vi "AssertInvisible.vi"(0 "VI Reference In":refnum<vi>, 1 "Label":string, 2 "delimiter (>>)":string=">>", 3 "Assert Only? (F)":bool, 5 "Control Path":string, 11 "Error In":errorcluster, 12 "Assert Interval(10 ms)":u32=10, 13 "Timeout(5 sec)":dbl=5.0) -> (4 "VI Reference Out":refnum<vi>, 6 "Asserted Value":bool caption="Asserted Value (Visible ?)", 15 "Error Out":errorcluster)   [LabVIEW 2016, in "Drona.lvlib" / "AssertControlProperty.lvlib" / "AssertControlVisible.lvlib"]
doc: "Asserts if the control is invisible.\n\nThe input control name is given as a string , incase of path, use delimiters inbetween the path.\nThis VI checks until the control is insvisible."
uses:
  AssertControlVisible.lvlib
  Get/GetControlRef/GetControlRefByPath.vi
  <vilib>/addons/_JKI Toolkits/Caraya/classes/Assert/Assert False.vi
  <vilib>/addons/_JKI Toolkits/Caraya/classes/Assert/Assert.lvclass
  Get/GetControlRef/GetControlRef.lvlib
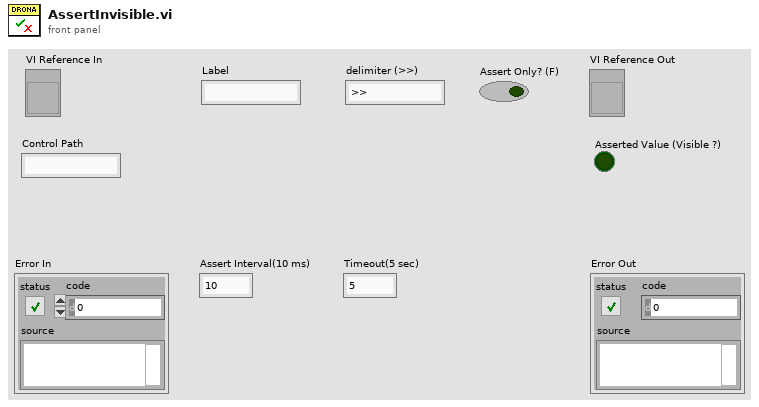
[diagram p1: front panel]
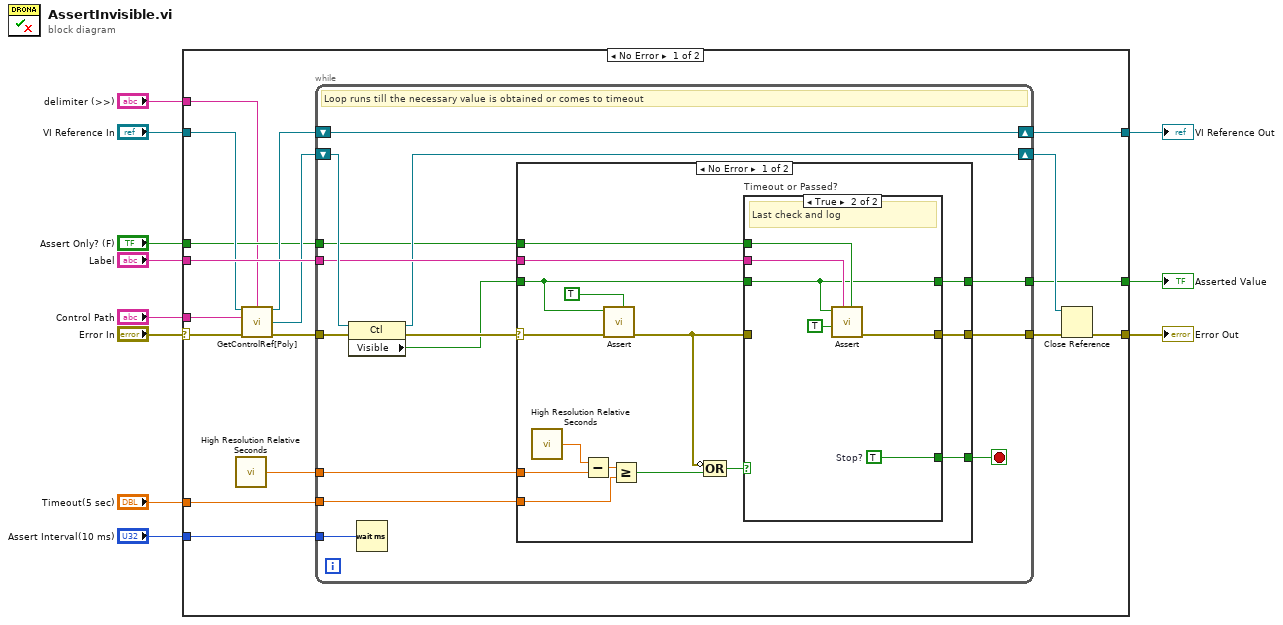
[diagram p0: block diagram]
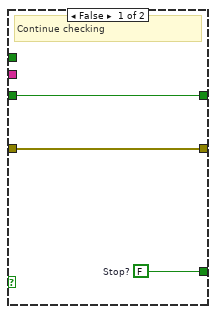
[diagram p2: hidden frame]
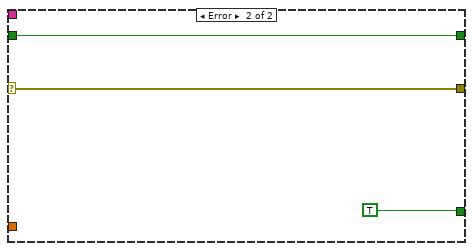
[diagram p3: hidden frame]
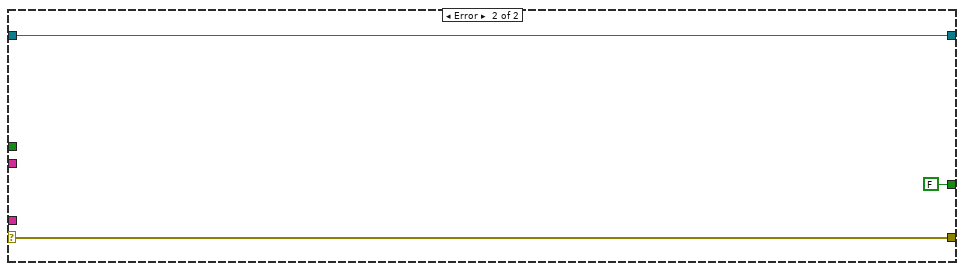
[diagram p4: hidden frame]
diagram:
  n1 = case shown="No Error" "Error In" {
    selector: "Error In" -> [w23 w72]
    tunnel: "Timeout(5 sec)" -> [w28 _]
    tunnel: [w27 w71] -> w10
    tunnel: [w17 w72] -> w9
    tunnel: "Assert Interval(10 ms)" -> [w25 _]
    tunnel: "Label" -> [w24 _]
    tunnel: "VI Reference In" -> [w22 w71]
    tunnel: "Control Path" -> [w12 _]
    tunnel: "delimiter (>>)" -> [w13 _]
    tunnel: "Assert Only? (F)" -> [w15 _]
    tunnel: [w14 FALSE ("Visible")] -> w1
    frame No Error {
      n2 = call <vilib>:"High Resolution Relative Seconds.vi"() -> ("relative seconds"=w21:dbl)
      n3 = call-poly "GetControlRef[Poly].vi"("VI Reference In"=w22, "delimiter (>>)"=w13, "Control Path"=w12, "error In"=w23) -> ("VI Reference Out"=w19:refnum<vi>, "Ctl Refnum"=w18:refnum<vi>, "error out"=w20:errorcluster)  [unwired: 9 in]
      n4 = while {
        tunnel: w28 -> [w41]
        tunnel: w21 -> [w42]
        tunnel: w20 -> [w36]
        tunnel: [w39] -> w26
        tunnel: w25 -> [w37]
        tunnel: w24 -> [w33]
        shift-right: [w34] -> w27
        shift-left: w19 -> [w34]
        shift-right: [w32] -> w16
        shift-left: w18 -> [w35]
        tunnel: w15 -> [w31]
        tunnel: [w29] -> w14
        stop <- w40 stop-if-true
        # "Loop runs till the necessary value is obtained or comes to timeout"
        n5 = property class="Ctl"(reference=w35, error in=w36) -> (reference out=w32:refnum<vi>, error out=w38:errorcluster, "Visible"=w30:bool)
        n6 = Wait (ms)(milliseconds to wait=w37) -> ()  [unwired: 1 out]
        n7 = case shown="No Error" w38 {
          selector: w38 -> [w53 w69]
          tunnel: w42 -> [w57 _]
          tunnel: w41 -> [w54 _]
          tunnel: [w46 TRUE] -> w40
          tunnel: [w47 w69] -> w39
          tunnel: w30 -> [w45 w67]
          tunnel: w33 -> [w52 _]
          tunnel: w31 -> [w44 _]
          tunnel: [w43 w67] -> w29
          frame No Error {
            n8 = call <vilib>:"High Resolution Relative Seconds.vi"() -> ("relative seconds"=w56:dbl)
            n9 = Subtract(x=w56, y=w57) -> (x-y=w55:dbl)
            n10 = call-poly <vilib>:"Assert.vi"("Assert Only? (F)"=TRUE, "error in (no error)"=w53, "False?"=w45) -> ("error out"=w50:errorcluster)  [unwired: 7 in, 1 out]
            n11 = Greater Or Equal?(x=w55, y=w54) -> (x >= y?=w51:bool)
            n12 = Compound Arithmetic op=OR(invert w50, w51) -> (w49:bool)
            n13 = case "Timeout or Passed?" shown="True" w49 {
              tunnel: w50 -> [w60 _]
              tunnel: w45 -> [w58 w62]
              tunnel: w52 -> [_ w66]
              tunnel: [w60 w65] -> w47
              tunnel: [w59 w64] -> w46
              tunnel: w44 -> [_ w63]
              tunnel: [w58 w62] -> w43
              frame False {
                w59 = FALSE  # Stop?
                # "Continue checking"
              }
              frame True {
                w64 = TRUE  # Stop?
                # "Last check and log"
                n14 = call-poly <vilib>:"Assert.vi"("Assert Only? (F)"=w63, "Label"=w66, "Register with caller test (F)"=TRUE, "False?"=w62) -> ("error out"=w65:errorcluster)  [unwired: 6 in, 1 out]
              }
            }
          }
          frame Error {
          }
        }
      }
      n15 = Close Reference(reference=w16, error in (no error)=w26) -> (error out=w17:errorcluster)
    }
    frame Error {
    }
  }
  "Error Out" <- w9
  "VI Reference Out" <- w10
  "Asserted Value" <- w1
